vi "LVClass_HasoField ctor.vi"(0 "HasoField in":refnum<class "HasoField.lvclass">, 1 "wavelenght nm":dbl, 2 "haso_config_file_path":path, 5 "HasoSlopes.lvclass":refnum<class "HasoSlopes.lvclass">, 7 "Phase.lvclass":refnum<class "Phase.lvclass">, 9 "radius_of_curvature _ mm":dbl, 11 "error in (no error)":errorcluster, 12 "oversampling_level":u8) -> (3 "wavelenght out":dbl, 4 "HasoField out":refnum<class "HasoField.lvclass">, 6 "HasoSlopes.lvclass dup":refnum<class "HasoSlopes.lvclass">, 15 "error out":errorcluster)   [LabVIEW 2020, in "HasoField.lvclass"]
doc: "HasoField constructor from HasoSlopes and phase.\n\n--------------------------------------------------------------------------------\n\n<B>HasoFieldIn </B> : Constant Pointer to HasoField object.\n<B>HasoFieldOut </B> : Constant Pointer to HasoField object.\n<B>haso_config_file_path </B> : Absolute path to Haso configuration file.\n<B>HasoSlopes </B> : HasoSlopes object.\n<B>Phase </B> : phase object.\n<B>radius_of_curvature </B> : Radius of curvature (mm).\n<B>wavelength </B> : Wavelenght of the source used to compute the HasoSlopes (nm).\n<B>oversampling_level </B> : Increment of oversampling level.\n<B>ErrorIn </B> : Error\n<B>ErrorOut </B> : Error\n\n--------------------------------------------------------------------------------"
uses:
  HasoField.lvclass
  HasoSlopes.lvclass
  Phase.lvclass
  Handle creation.ctl
  HasoField.lvclass/HasoField.ctl
  LVClasse_Phase Read SurfaceFloatWithPupil.vi
  LVClass_HasoSlopes Read HasoSlopes _ property.vi
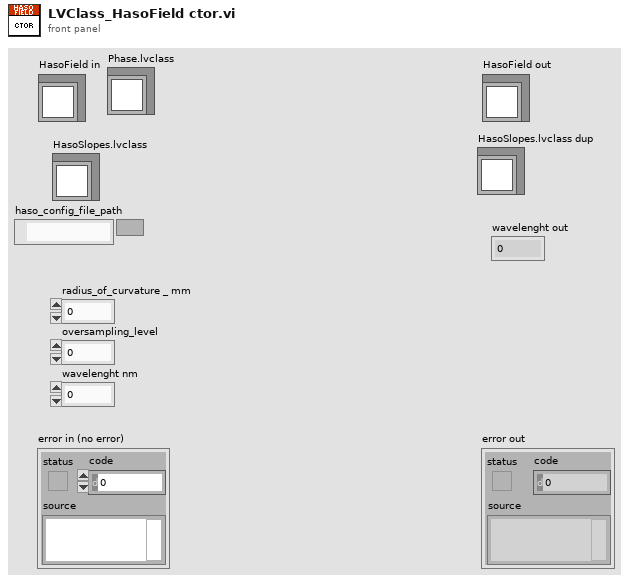
[diagram p1: front panel]
types:
  T1 = typedef "Handle creation.ctl" = enum16{"By ctor", "By write function"}
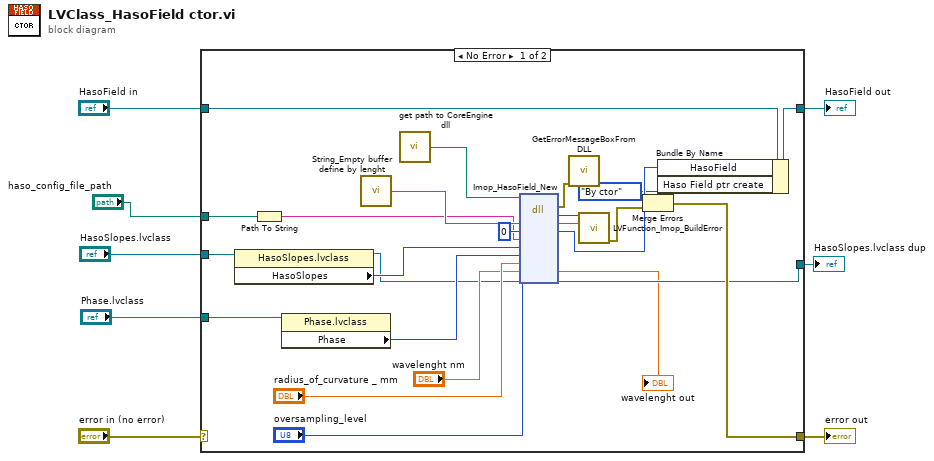
[diagram p0: block diagram]
diagram:
  n1 = case shown="No Error" "error in (no error)" {
    selector: "error in (no error)" -> [_ w35]
    tunnel: [w23 w35] -> w7
    tunnel: [w16 w34] -> w5
    tunnel: "HasoField in" -> [w17 w34]
    tunnel: "HasoSlopes.lvclass" -> [w25 w33]
    tunnel: "Phase.lvclass" -> [w24 _]
    tunnel: [w12 w33] -> w3
    tunnel: "haso_config_file_path" -> [w9 _]
    frame No Error {
      n2 = property class="HasoSlopes.lvclass"(reference=w25) -> (reference out=w12:refnum<class "HasoSlopes.lvclass">, "HasoSlopes"=w22:i32)  [unwired: 1 in, 1 out]
      n3 = Path To String(path=w9) -> (string=w10:string)
      n4 = property class="Phase.lvclass"(reference=w24) -> ("Phase"=w21:i32)  [unwired: 1 in, 2 out]
      n5 = call "String_Empty buffer define by lenght.vi"() -> ("Empty buffer"=w32:string)  [unwired: 1 in]
      n6 = call "get path to CoreEngine dll.vi"() -> ("path to c_interface_vc100.dll"=w29:path)  [unwired: 12 in, 3 out]
      n7 = dll-call lib="D:/soft/HASO_v3/SVN_trunk/ImOpCoreEngine4_LV2011/DLLs/c_interface_vc100.dll" fn="Imop_HasoField_New"(path in=w29, "message"=w32, "hasofield"=0, "haso_config_file_path"=w10, "HasoSlopes"=w22, "Phase"=w21, "radius_of_curvature"="radius_of_curvature _ mm", "wavelenght"="wavelenght nm", "oversampling_level"="oversampling_level") -> (error out=w28:errorcluster, "return type"=w30:i32, "message"=w31:string, "hasofield"=w15:i32, "wavelenght"=→"wavelenght out":dbl)  [unwired: 7 in, 1 out]
      n8 = call "GetErrorMessageBoxFromDLL.vi"("error IN"=w28) -> ("error OUT"=w27:errorcluster)  [unwired: 10 in]
      n9 = call "LVFunction_Imop_BuildError.vi"("code"=w30, "String to Prepend to source (\"\")"=w31) -> ("error out"=w26:errorcluster)  [unwired: 13 in]
      n10 = Merge Errors(w27, w26) -> (w23:errorcluster)
      n11 = Bundle By Name(cluster=w17, "HasoField"=w15, "Haso Field ptr create"=Handle_creation."By ctor") -> (w16:refnum<class "HasoField.lvclass">)
    }
    frame Error {
    }
  }
  "error out" <- w7
  "HasoField out" <- w5
  "HasoSlopes.lvclass dup" <- w3
